vi "setup-488.vi"() -> ()   [LabVIEW 2012]
uses:
  <vilib>/DAQmx/write.llb/DAQmx Write (Analog DBL 1Chan 1Samp).vi
  <vilib>/DAQmx/create/channels.llb/DAQmx Create Channel (AO-Voltage-Basic).vi
  <vilib>/DAQmx/configure/trigger.llb/DAQmx Start Trigger (Digital Edge).vi
  <vilib>/DAQmx/miscellaneous.llb/DAQmx Fill In Error Info.vi
  <resource>/objmgr/daqmx.rc
panel:
  in  "error in":errorcluster
  in  "physical channels":tag="Dev2/ao1"
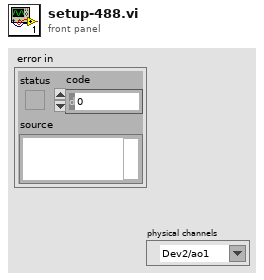
[diagram p1: front panel]
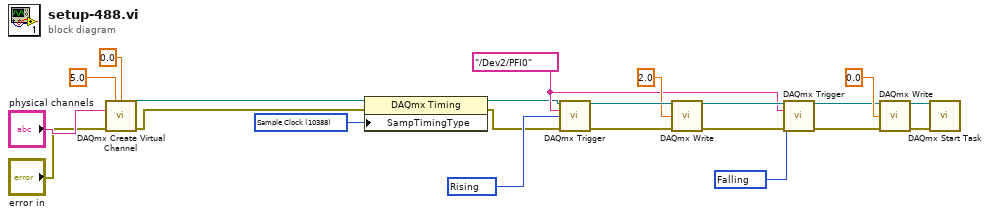
[diagram p0: block diagram]
diagram:
  w1 = 10388 items=["Sample Clock"=10388, "Burst Handshake"=12548, "Handshake"=10389, "Implicit"=10451, "On Demand"=10390, "Change Detection"=12504, "Pipelined Sample Clock"=14668] ("SampTimingType")
  w14 = 10171 items=["Rising"=10280, "Falling"=10171] ("edge")
  w11 = tag "/Dev2/PFI0" ("source")
  w18 = 10280 items=["Rising"=10280, "Falling"=10171] ("edge")
  n1 = call-poly <vilib>:"DAQmx Create Virtual Channel.vi"("maximum value"=5.0, "minimum value"=0.0, "physical channels"="physical channels", "error in"="error in") -> ("task out"=w2:refnum<k21>, "error out"=w3:errorcluster)  [unwired: 10 in]
  n2 = property class="DAQmx Timing"(reference=w2, error in=w3, "SampTimingType"=w1) -> (reference out=w4:refnum<k21>, error out=w5:errorcluster)
  n3 = call-poly <vilib>:"DAQmx Trigger.vi"("task/channels in"=w4, "source"=w11, "edge"=w18, "error in"=w5) -> ("task out"=w16:refnum<k21>, "error out"=w17:errorcluster)  [unwired: 10 in]
  n4 = call-poly <vilib>:"DAQmx Write.vi"("task/channels in"=w16, "data"=2.0, "error in"=w17) -> ("task out"=w12:refnum<k21>, "error out"=w13:errorcluster)  [unwired: 10 in, 1 out]
  n5 = call-poly <vilib>:"DAQmx Trigger.vi"("task/channels in"=w12, "source"=w11, "edge"=w14, "error in"=w13) -> ("task out"=w9:refnum<k21>, "error out"=w8:errorcluster)  [unwired: 10 in]
  n6 = call-poly <vilib>:"DAQmx Write.vi"("task/channels in"=w9, "data"=0.0, "error in"=w8) -> ("task out"=w6:refnum<k21>, "error out"=w7:errorcluster)  [unwired: 10 in, 1 out]
  n7 = call <vilib>:"DAQmx Start Task.vi"("task/channels in"=w6, "error in"=w7) -> ()  [unwired: 12 in, 2 out]
